vi "Uint8Array Destroy.vi"(8 "error in (no error)":errorcluster, 11 "Uint8Array DVR in":refnum<data-value>) -> (0 "error out":errorcluster)   [LabVIEW 2012, in "MDSplus.lvlib"]
uses:
  <vilib>/MDSplus/Library/MDSplus.lvlib
  <vilib>/MDSplus/Classes/Data_Class/Array_Class/Uint8Array_Class/Uint8Array.lvclass
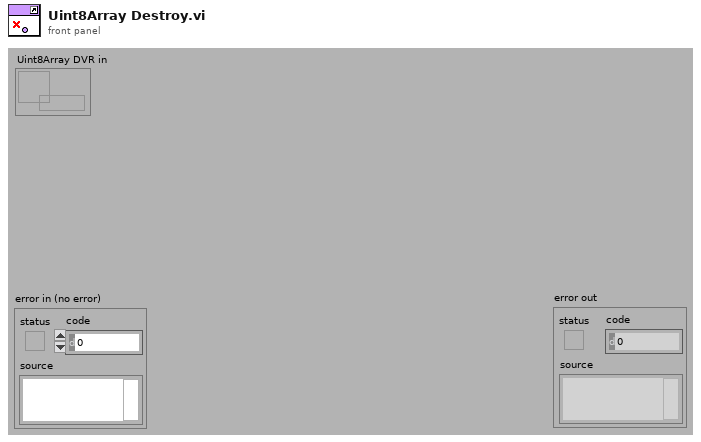
[diagram p1: front panel]
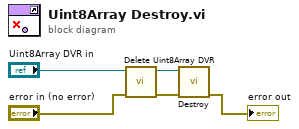
[diagram p0: block diagram]
diagram:
  n1 = call <vilib>:"Delete Uint8Array DVR.vi"("error in (no error)"="error in (no error)", "Uint8Array DVR in"="Uint8Array DVR in") -> ("error out"=w2:errorcluster, "Uint8Array out"=w3:refnum<class "Uint8Array.lvclass">)  [unwired: 8 in]
  n2 = call-dynamic "Destroy.vi"("error in (no error)"=w2, "Uint8Array in"=w3) -> ("error out"=→"error out":errorcluster)  [unwired: 9 in]
